vi "NPSH3%.vi"(8 "% caduta":dbl=3.0 format="%#_13g", 9 "Pto in corso":i32=1, 10 "indici":T1, 11 "TABELLA MISURE":string[][](array[string])) -> (0 "Npsh3%":dbl, 1 "NPSH interp":cluster{dbl[], dbl[]}, 2 "Htot-3%":dbl, 3 "TABELLA MISURE OUT":string[][](array[string]))   [LabVIEW 2019]
uses:
  TypeDef/Indici.ctl
panel:
  out "XY Graph":cluster{dbl[], dbl[]}[](graph)
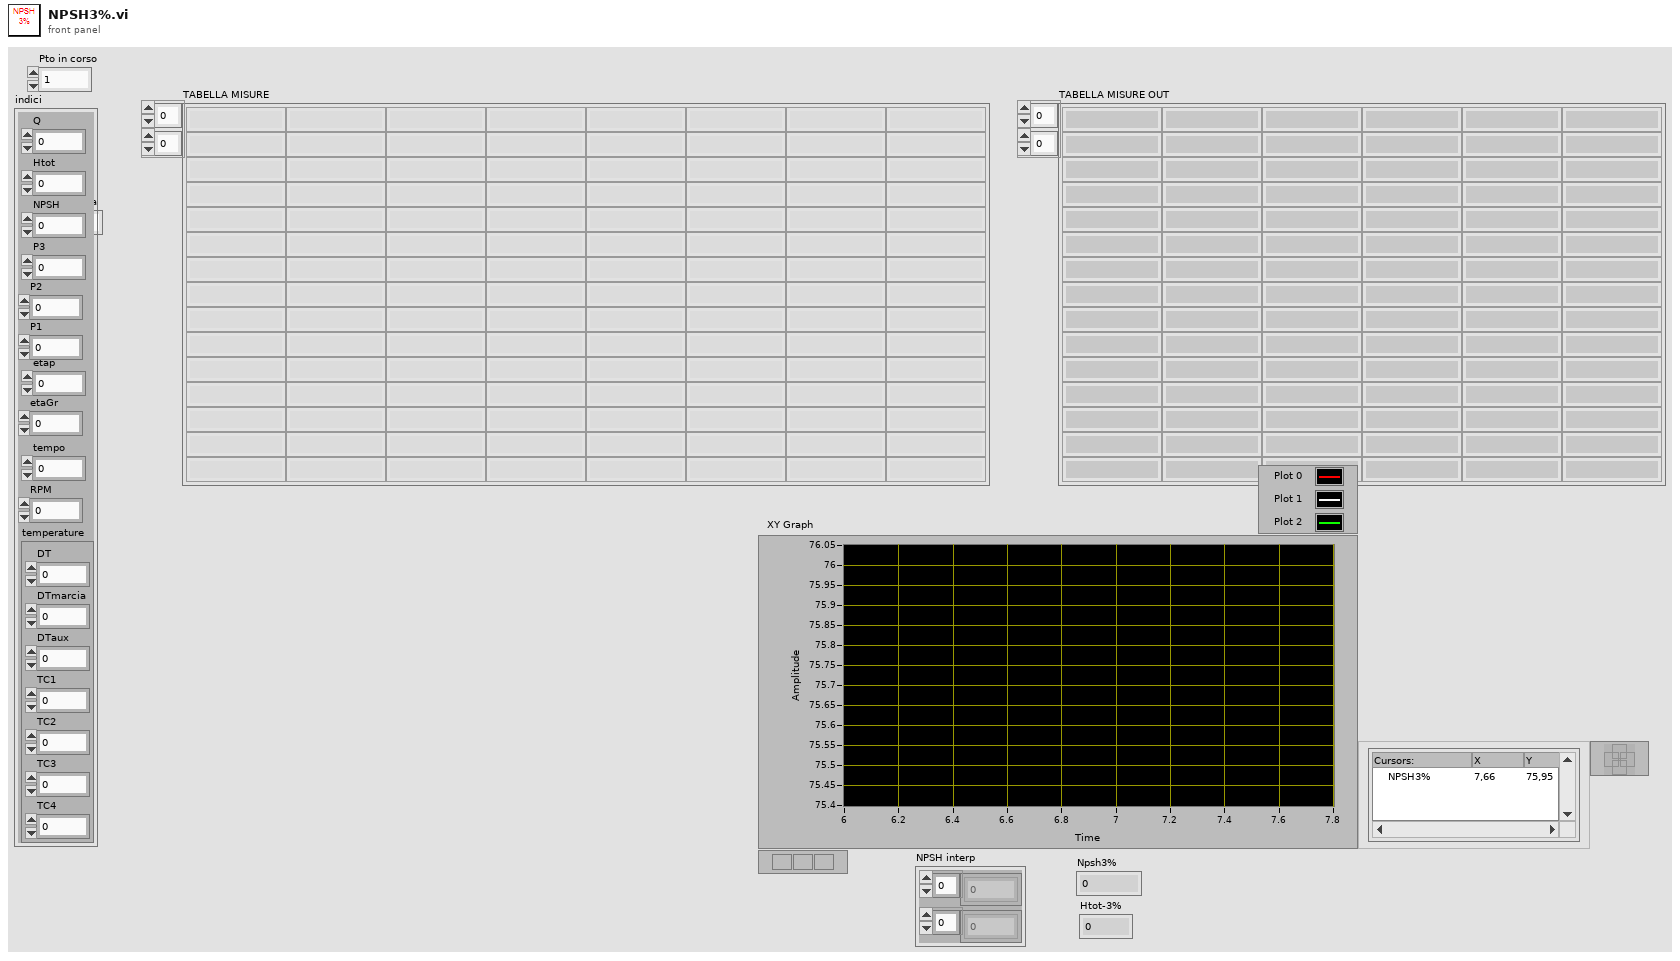
[diagram p1: front panel]
types:
  T1 = typedef "Indici.ctl" = cluster{"Q":i32, "Htot":i32, "NPSH":i32, "P3":i32, "etap":i32, "temperature":cluster{"DT":i32, "DTmarcia":i32, "DTaux":i32, "TC1":i32, "TC2":i32, "TC3":i32, "TC4":i32}, "tempo":i32, "P2":i32, "P1":i32, "etaGr":i32, "RPM":i32}
  T2 = cluster{"punto":i32, "cluster":cluster{"index":i32, "length":i32}}[]
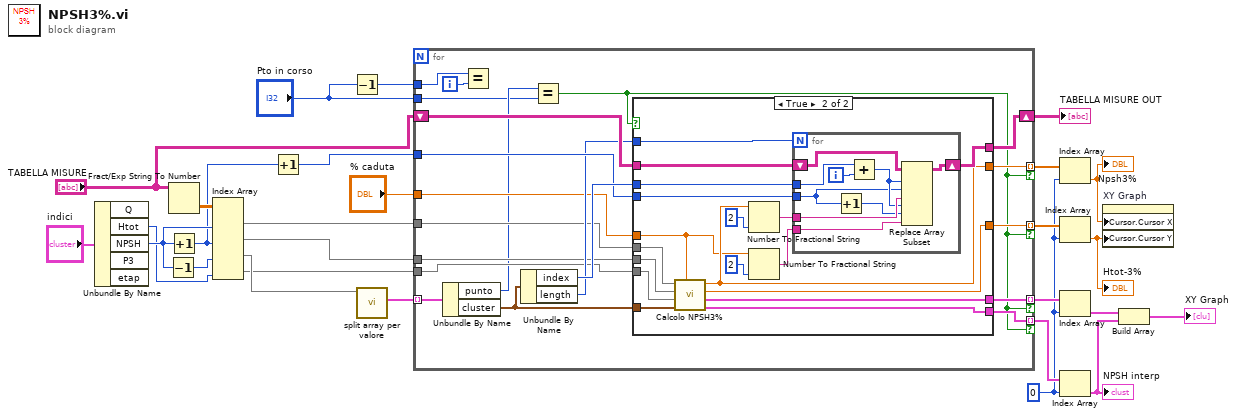
[diagram p0: block diagram]
diagram:
  w5 = 0 ("index")
  n1 = Unbundle By Name("indici") -> ("Htot"=w17:i32, "NPSH"=w26:i32)  [unwired: 3 out]
  n2 = Decrement(x=w26) -> (x-1=w25:i32)
  n3 = Fract/Exp String To Number(string="TABELLA MISURE") -> (number=w27:dbl[][])  [unwired: 3 in, 1 out]
  n4 = Increment(x=w26) -> (x+1=w22:i32)
  n5 = Index Array(array=w27, index (col) #1=w26, index (col) #2=w22, index (col) #3=w25, index (col) #4=w17) -> (element #1=w18:dbl[], element #2=w16:dbl[], element #3=w24:dbl[], element #4=w15:dbl[])  [unwired: 4 in]
  n6 = Increment(x=w22) -> (x+1=w21:i32)
  n7 = Decrement(x="Pto in corso") -> (x-1=w14:i32)
  n8 = call <userlib>:"split array per valore.vi"("Array"=w24) -> ("sorted array"=w2:T2)  [unwired: 10 in]
  n9 = for {
    tunnel: w2 -> [w33] mode=indexing
    tunnel: w16 -> [w41]
    tunnel: w18 -> [w42]
    shift-right: [w43] -> w20
    shift-left: "TABELLA MISURE" -> [w47]
    tunnel: w21 -> [w45]
    tunnel: w15 -> [w40]
    tunnel: [w39] -> w13 mode=indexing if=w28
    tunnel: [w38] -> w12 mode=indexing if=w28
    tunnel: [w37] -> w11 mode=indexing if=w28
    tunnel: [w36] -> w10 mode=indexing if=w28
    tunnel: w14 -> [w35]
    tunnel: "% caduta" -> [w34]
    tunnel: "Pto in corso" -> [w29]
    i -> [w30]
    n10 = Unbundle By Name(w33) -> ("punto"=w31:i32, "cluster"=w32:cluster{"index":i32, "length":i32})
    n11 = Equal?(x=w35, y=w30) -> ()  [unwired: 1 out]
    n12 = Unbundle By Name(w32) -> ("index"=w46:i32, "length"=w44:i32)
    n13 = Equal?(x=w31, y=w29) -> (x = y?=w28:bool)
    n14 = case shown="True" w28 {
      tunnel: w47 -> [w48 w66]
      tunnel: w46 -> [_ w65]
      tunnel: w45 -> [_ w64]
      tunnel: w44 -> [_ w63]
      tunnel: [w48 w60] -> w43
      tunnel: w42 -> [_ w59]
      tunnel: w41 -> [_ w58]
      tunnel: w40 -> [_ w57]
      tunnel: [_ w56] -> w39
      tunnel: [_ w55] -> w38
      tunnel: [_ w54] -> w37
      tunnel: [_ w53] -> w36
      tunnel: w34 -> [_ w51]
      tunnel: w32 -> [_ w49]
      frame False {
      }
      frame True {
        n15 = call "Calcolo NPSH3%.vi"("% caduta"=w51, "Cluster in"=w49, "Htot"=w57, "Htot ref[m]"=w58, "npsh"=w59) -> ("Graph interp"=w53:cluster{dbl[], dbl[]}, "Graph"=w54:cluster{dbl[], dbl[]}, "Htot-3%"=w55:dbl, "Npsh3%"=w56:dbl)  [unwired: 3 in]
        n16 = Number To Fractional String(number=w56, precision (6)=i16 2) -> (F-format string=w61:string)  [unwired: 2 in]
        n17 = Number To Fractional String(number=w51, precision (6)=i16 2) -> (F-format string=w50:string)  [unwired: 2 in]
        n18 = for {
          N: w63 -> [_]
          tunnel: w65 -> [w74]
          shift-right: [w71] -> w60
          shift-left: w66 -> [w75]
          tunnel: w64 -> [w69]
          tunnel: w61 -> [w72]
          tunnel: w50 -> [w67]
          i -> [w73]
          n19 = Increment(x=w69) -> (x+1=w68:i32)
          n20 = Add(x=w74, y=w73) -> (x+y=w70:i32)
          n21 = Replace Array Subset(array=w75, new element #1=w72, index (row) #1=w70, index (col) #1=w69, new element #2=w67, index (row) #2=w70, index (col) #2=w68) -> (w71:string[][])
        }
      }
    }
  }
  "TABELLA MISURE OUT" <- w20
  n22 = Index Array(array=w13, index=w5) -> (element=w6:dbl)
  "Npsh3%" <- w6
  n23 = Index Array(array=w12, index=w5) -> (element=w9:dbl)
  "Htot-3%" <- w9
  n24 = Index Array(array=w11, index=w5) -> (element=w8:cluster{dbl[], dbl[]})
  n25 = Index Array(array=w10, index=w5) -> (element=w7:cluster{dbl[], dbl[]})
  "NPSH interp" <- w7
  n26 = property on="XY Graph" class="XYGraph (strict)"("Cursor.Cursor X"=w6, "Cursor.Cursor Y"=w9) -> ()  [unwired: 2 in, 2 out]
  n27 = Build Array(w8, w7) -> (→"XY Graph":cluster{dbl[], dbl[]}[])
